vi "Open Sensor Sessions.vi"() -> (0 "Motor out":refnum<visa-resource-name>, 1 "Relay out":refnum<visa-resource-name>, 3 "Sensor Sessions":T2)   [LabVIEW 2011]
uses:
  <vilib>/vision/Image Controls.llb/IMAQ Image.ctl
  <instrlib>/Hokuyo URG Series/Public/Initialize-Standard.vi
  <instrlib>/Ocean Server OS4000/Ocean Server OS4000.lvlib
  <instrlib>/Hokuyo URG Series/Hokuyo URG Series.lvlib
  <instrlib>/u-blox 5 Series/u-blox 5 Series.lvlib
panel:
  in  "Relay COM":refnum<visa-resource-name>
  in  "Motor COM":refnum<visa-resource-name>
  in  "GPS COM":refnum<visa-resource-name>
  in  "LineCam COM":refnum<visa-resource-name>
  in  "LIDAR COM":refnum<visa-resource-name>
  in  "Compass COM":refnum<visa-resource-name>
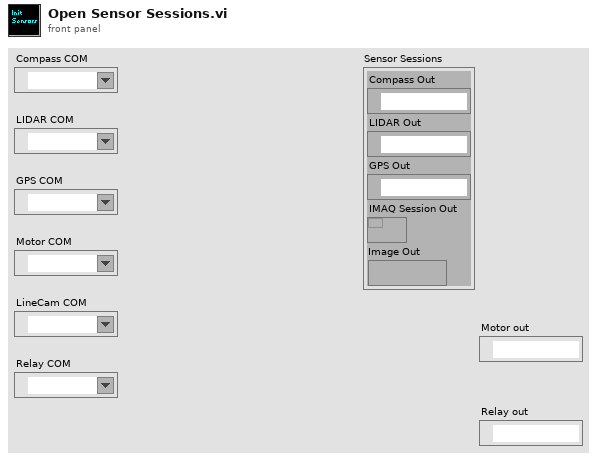
[diagram p1: front panel]
types:
  T1 = typedef "IMAQ Image.ctl" = refnum<image>
  T2 = cluster{"Compass Out":refnum<visa-resource-name>, "LIDAR Out":refnum<visa-resource-name>, "GPS Out":refnum<visa-resource-name>, "IMAQ Session Out":refnum<k11>, "Image Out":T1}
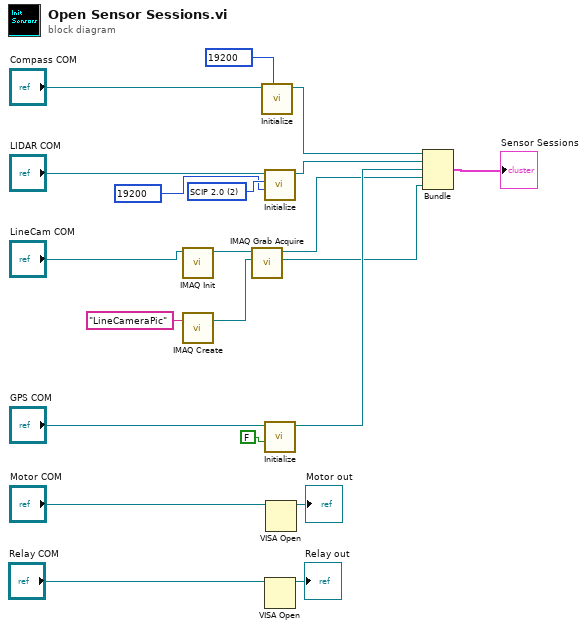
[diagram p0: block diagram]
diagram:
  w11 = u32 19200 items=["4800"=4800, "9600"=9600, "14400"=14400, "19200"=19200, "38400"=38400, "57600"=57600, "115200"=115200] ("Baud Rate")
  w12 = u32 19200 items=["19200"=19200, "57600"=57600, "115200"=115200, "250000"=250000, "500000"=500000, "750000"=750000] ("Serial Configuration (19200 : 19200 Baud)")
  w13 = u32 2 items=["Convert to Latest", "SCIP 1.1", "SCIP 2.0"] ("Protocol (2: SCIP 2.0)")
  n1 = call <vilib>:"IMAQ Init.vi"("Interface Name"="LineCam COM") -> ("IMAQ Session Out"=w8:refnum<k11>)  [unwired: 9 in, 1 out]
  n2 = call "IMAQ Create"("Image Name"="LineCameraPic") -> ("New Image"=w6:T1)  [unwired: 4 in, 1 out]
  n3 = call <vilib>:"IMAQ Grab Acquire.vi"("Image In"=w6, "IMAQ Session In"=w8) -> ("Image Out"=w2:T1, "IMAQ Session Out"=w3:refnum<k11>)  [unwired: 6 in, 2 out]
  n4 = call <instrlib>:"Initialize.vi"("Baud Rate"=w11, "VISA resource name"="Compass COM") -> ("Compass Out"=w16:refnum<visa-resource-name>)  [unwired: 8 in, 1 out]
  n5 = call-poly <instrlib>:"Initialize.vi"("Serial Configuration (19200 : 19200 Baud)"=w12, "Protocol (2: SCIP 2.0)"=w13, "VISA resource name"="LIDAR COM") -> ("LIDAR Out"=w14:refnum<visa-resource-name>)  [unwired: 7 in, 1 out]
  n6 = call <instrlib>:"Initialize.vi"("Reset (False)"=FALSE, "VISA resource name"="GPS COM") -> ("GPS Out"=w4:refnum<visa-resource-name>)  [unwired: 8 in, 1 out]
  n7 = VISA Open(VISA resource name="Relay COM") -> (VISA resource name=→"Relay out":refnum<visa-resource-name>)  [unwired: 4 in, 1 out]
  n8 = VISA Open(VISA resource name="Motor COM") -> (VISA resource name=→"Motor out":refnum<visa-resource-name>)  [unwired: 4 in, 1 out]
  n9 = Bundle("Compass Out"=w16, "LIDAR Out"=w14, "GPS Out"=w4, "IMAQ Session Out"=w3, "Image Out"=w2) -> (→"Sensor Sessions":T2)  [unwired: 1 in]
